vi "santhos bro practice.vi"() -> ()   [LabVIEW 2021]
panel:
  in  "Delete":bool
  out "Array 2":string[][](array[string])
  in  "File path (Use dialog) 2":path
  in  "Read":bool
  in  "Write":bool
  in  "Array":string[][](array[string])
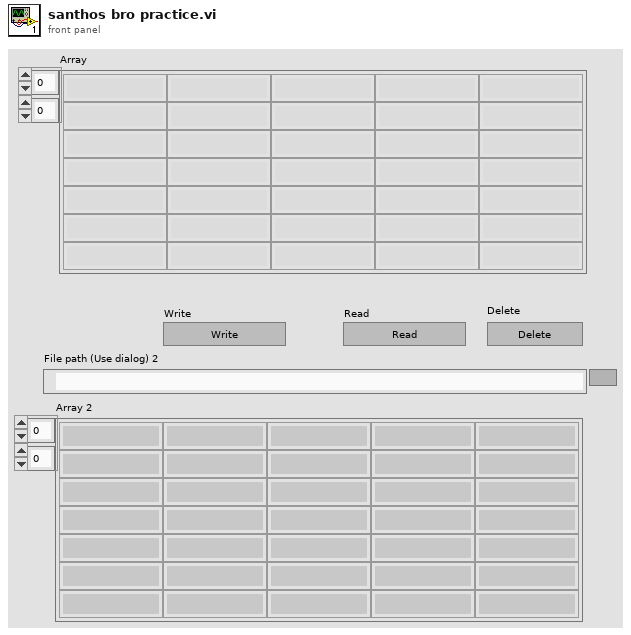
[diagram p1: front panel]
types:
  T1 = enum16{"open", "replace", "create", "open or create", "replace or create", "replace or create with confirmation"}
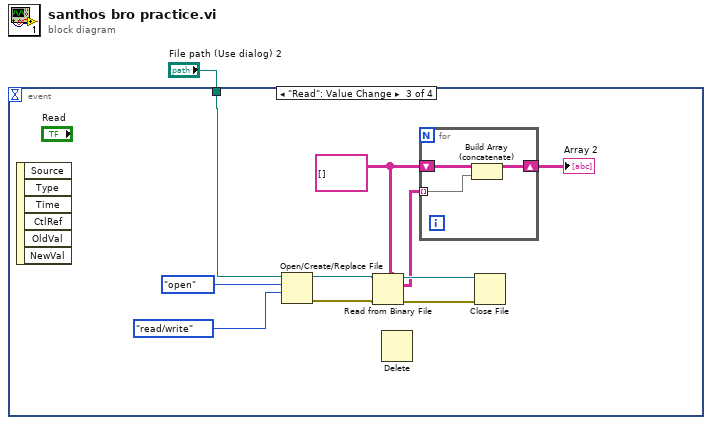
[diagram p0: block diagram]
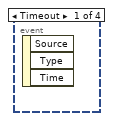
[diagram p2: hidden frame]
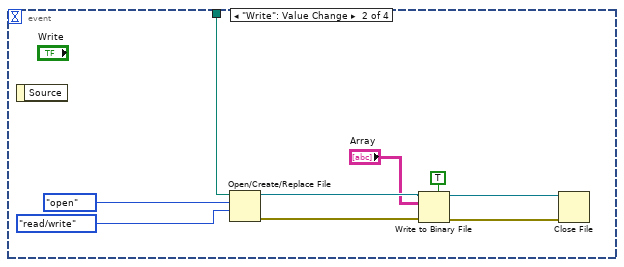
[diagram p3: hidden frame]
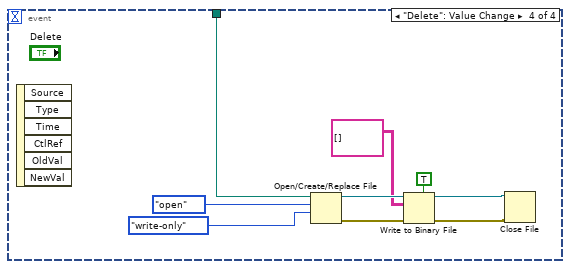
[diagram p4: hidden frame]
diagram:
  n1 = event shown="[2] \"Read\": Value Change" {
    selector: _ -> [_ _ _ _]
    dyn-events: _ -> [_ _ _ _]
    timeout: _ -> [_ _ _ _]
    tunnel: "File path (Use dialog) 2" -> [_ w2 w12 w24]
    event Timeout {
      n2 = event-data() -> ()  [unwired: 1 in, 3 out]
    }
    event "Write": Value Change {
      n3 = event-data() -> ()  [unwired: 1 in, 1 out]
      n4 = Open/Create/Replace File(file path (use dialog)=w2, operation (0:open)=T1."open", access (0:read/write)=enum16{"read/write", "read-only", "write-only"}."read/write") -> (refnum out=w10:refnum<file>, error out=w8:errorcluster)  [unwired: 3 in, 1 out]
      n5 = Write to Binary File(file (use dialog)=w10, data="Array", error in=w8, 5:TRUE) -> (refnum out=w9:refnum<file>, error out=w7:errorcluster)  [unwired: 2 in, 1 out]
      n6 = Close File(refnum=w9, error in=w7) -> ()  [unwired: 2 out]
    }
    event "Read": Value Change {
      w13 = string[][] [] ("Array 2")
      n7 = event-data() -> ()  [unwired: 1 in, 6 out]
      n8 = Open/Create/Replace File(file path (use dialog)=w12, operation (0:open)=T1."open", access (0:read/write)=enum16{"read/write", "read-only", "write-only"}."read/write") -> (refnum out=w11:refnum<file>, error out=w19:errorcluster)  [unwired: 3 in, 1 out]
      n9 = Read from Binary File(5:w13, 8:w19, 11:w11) -> (0:w18:errorcluster, 2:w15:string[][], 3:w20:refnum<file>)  [unwired: 3 in, 1 out]
      n10 = Delete() -> ()  [unwired: 5 in, 3 out]
      n11 = for {
        tunnel: w15 -> [w23] mode=indexing
        shift-right: [w21] -> w14
        shift-left: w13 -> [w22]
        n12 = Build Array (concatenate)(w22, w23) -> (w21:string[][])
      }
      "Array 2" <- w14
      n13 = Close File(refnum=w20, error in=w18) -> ()  [unwired: 2 out]
    }
    event "Delete": Value Change {
      n14 = event-data() -> ()  [unwired: 1 in, 6 out]
      n15 = Open/Create/Replace File(file path (use dialog)=w24, operation (0:open)=T1."open", access (0:read/write)=enum16{"read/write", "read-only", "write-only"}."write-only") -> (refnum out=w32:refnum<file>, error out=w30:errorcluster)  [unwired: 3 in, 1 out]
      n16 = Write to Binary File(file (use dialog)=w32, data=string[][] [] ("text"), error in=w30, 5:TRUE ("prepend array or string size? (T)")) -> (refnum out=w31:refnum<file>, error out=w29:errorcluster)  [unwired: 2 in, 1 out]
      n17 = Close File(refnum=w31, error in=w29) -> ()  [unwired: 2 out]
    }
  }
